vi "Open Excel Ref.vi"(8 "error in":errorcluster) -> (0 "error out":errorcluster, 3 "excelRefs out":T1)   [LabVIEW 2020]
uses:
  Controls/excelRefContainer.ctl
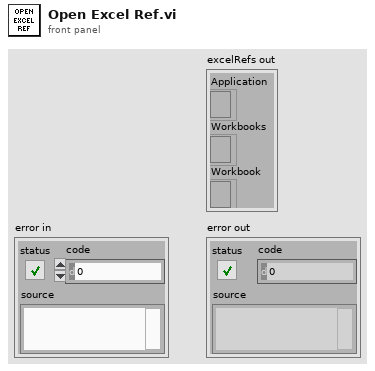
[diagram p1: front panel]
types:
  T1 = typedef "excelRefContainer.ctl" = cluster{"Application":refnum<k7>, "Workbooks":refnum<k7>, "Workbook":refnum<k7>}
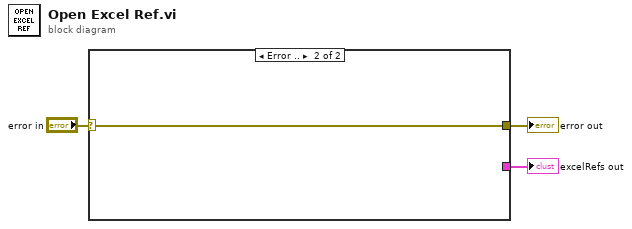
[diagram p0: block diagram]
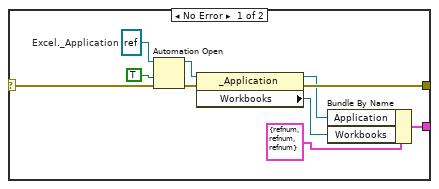
[diagram p2: hidden frame]
diagram:
  n1 = case shown="Error .." "error in" {
    selector: "error in" -> [w9 w14]
    tunnel: [w8 w14] -> w2
    tunnel: [w6 _] -> w1
    frame No Error {
      w13 = refnum<k7> refnum  # Excel._Application
      n2 = Automation Open(error in (no error)=w9, Automation Refnum=w13, 9:TRUE ("open new instance (false)")) -> (Automation Refnum=w11:refnum<k7>, error out=w12:errorcluster)  [unwired: 1 in]
      n3 = property class="_Application"(reference=w11, error in=w12) -> (reference out=w5:refnum<k7>, error out=w8:errorcluster, "Workbooks"=w4:refnum<k7>)
      n4 = Bundle By Name(cluster=T1 {"Application"=refnum, "Workbooks"=refnum, "Workbook"=refnum}, "Application"=w5, "Workbooks"=w4) -> (w6:T1)
    }
    frame Error {
    }
  }
  "error out" <- w2
  "excelRefs out" <- w1
